vi "SpeedControl.vi"(0 "XPos":refnum<vi>, 1 "CurrentX":refnum<vi>, 2 "YPos":refnum<vi>, 3 "CurrentY":refnum<vi>, 4 "SelectPol":refnum<vi>, 5 "错误输入（无错误）":errorcluster) -> (14 "1轴速度":i32, 15 "2轴速度":i32, 19 "错误输出":errorcluster)   [LabVIEW 2011]
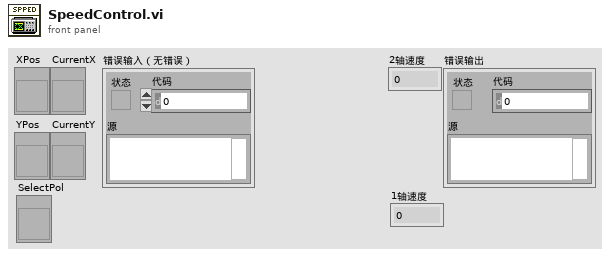
[diagram p1: front panel]
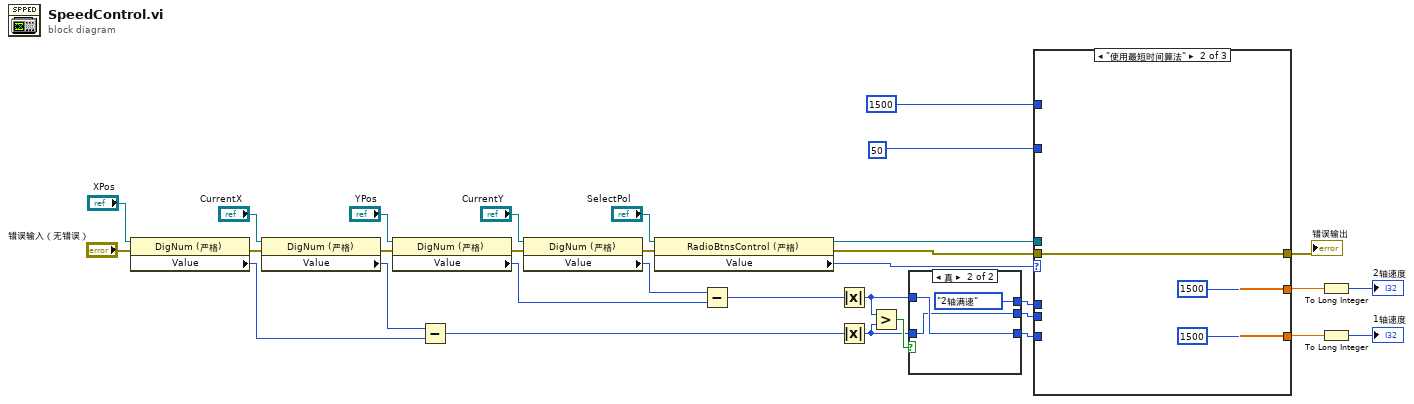
[diagram p0: block diagram]
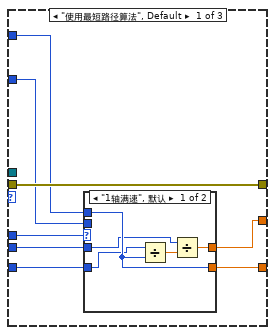
[diagram p2: hidden frame]
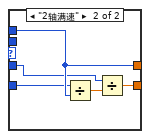
[diagram p3: hidden frame]
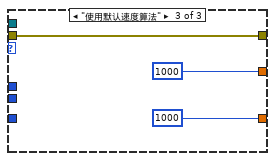
[diagram p4: hidden frame]
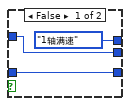
[diagram p5: hidden frame]
diagram:
  n1 = property on="属性节点" class="DigNum (严格)"(reference="XPos", error in="错误输入（无错误）") -> (error out=w32:errorcluster, "Value"=w22:i32)  [unwired: 1 out]
  n2 = property on="属性节点" class="DigNum (严格)"(reference="CurrentX", error in=w32) -> (error out=w31:errorcluster, "Value"=w21:i32)  [unwired: 1 out]
  n3 = property on="属性节点" class="DigNum (严格)"(reference="YPos", error in=w31) -> (error out=w30:errorcluster, "Value"=w18:i32)  [unwired: 1 out]
  n4 = Subtract(x=w21, y=w22) -> (x-y=w20:i32)
  n5 = property on="属性节点" class="DigNum (严格)"(reference="CurrentY", error in=w30) -> (error out=w24:errorcluster, "Value"=w17:i32)  [unwired: 1 out]
  n6 = property class="RadioBtnsControl (严格)"(reference="SelectPol", error in=w24) -> (reference out=w12:refnum<vi>, error out=w11:errorcluster, "Value"=w13:enum32{"使用最短路径算法", "使用最短时间算法", "使用默认速度算法"})
  n7 = Subtract(x=w17, y=w18) -> (x-y=w19:i32)
  n8 = Absolute Value(x=w19) -> (abs(x)=w15:i32)
  n9 = Absolute Value(x=w20) -> (abs(x)=w14:i32)
  n10 = Greater?(x=w15, y=w14) -> (0:w16:bool)
  n11 = case shown="真" w16 {
    tunnel: w15 -> [w35 w38]
    tunnel: w14 -> [w34 w37]
    tunnel: [w34 w38] -> w10
    tunnel: [w35 w37] -> w9
    tunnel: [enum16{"1轴满速", "2轴满速"}."1轴满速" enum16{"1轴满速", "2轴满速"}."2轴满速"] -> w8
    frame False {
    }
    frame True {
    }
  }
  n12 = case shown="\"使用最短时间算法\"" w13 {
    tunnel: w12 -> [_ _ _]
    tunnel: w11 -> [w46 w57 w60]
    tunnel: [w44 1500 1000] -> w7
    tunnel: [w41 1500 1000] -> w6
    tunnel: w10 -> [w43 _ _]
    tunnel: w9 -> [w42 _ _]
    tunnel: w8 -> [w45 _ _]
    tunnel: [w46 w57 w60] -> w5
    tunnel: 1500 -> [w40 _ _]
    tunnel: 50 -> [w39 _ _]
    frame "使用最短路径算法", Default {
      n13 = case shown="\"1轴满速\", 默认" w45 {
        tunnel: [w49 w55] -> w44
        tunnel: w43 -> [w47 w52]
        tunnel: w42 -> [w48 w53]
        tunnel: [w50 w54] -> w41
        tunnel: w40 -> [w49 w54]
        tunnel: w39 -> [_ _]
        frame "1轴满速", Default {
          n14 = Divide(x=w47, y=w49) -> (x/y=w51:dbl)
          n15 = Divide(x=w48, y=w51) -> (x/y=w50:dbl)
        }
        frame "2轴满速" {
          n16 = Divide(x=w52, y=w54) -> (x/y=w56:dbl)
          n17 = Divide(x=w53, y=w56) -> (x/y=w55:dbl)
        }
      }
    }
    frame "使用最短时间算法" {
    }
    frame "使用默认速度算法" {
    }
  }
  "错误输出" <- w5
  n18 = To Long Integer(number=w6) -> (32bit integer=→"2轴速度":i32)
  n19 = To Long Integer(number=w7) -> (32bit integer=→"1轴速度":i32)
